vi "SDF Small Gasifier RT - Alarms.vi"() -> ()   [LabVIEW 2013]
uses:
  <vilib>/NI/Current Value Table/DataTypes/Boolean_Read.vi
  <vilib>/NI/Current Value Table/DataTypes/Double_Read.vi
  <vilib>/NI/Current Value Table/DataTypes/Boolean_Write.vi
  <vilib>/NI/Current Value Table/Type to Enum.vi
  <vilib>/NI/Current Value Table/DataTypes/Boolean_Type To Enum.vi
  <vilib>/NI/Current Value Table/DataTypes/Double_Type To Enum.vi
  <vilib>/NI/Current Value Table/FGVs/CVT Globals.vi
  <vilib>/NI/Current Value Table/FGVs/Tag Memory.vi
  <vilib>/NI/Current Value Table/Memory Block.vi
  <vilib>/NI/Current Value Table/DataTypes/Boolean_Memory Block.vi
  <vilib>/NI/Current Value Table/DataTypes/Double_Memory Block.vi
  <vilib>/NI/Current Value Table/Current Value Table.lvlib
panel:
  in  "Stop":bool
  out "Index":i32
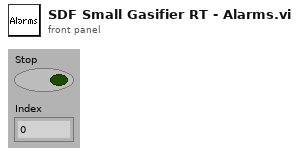
[diagram p1: front panel]
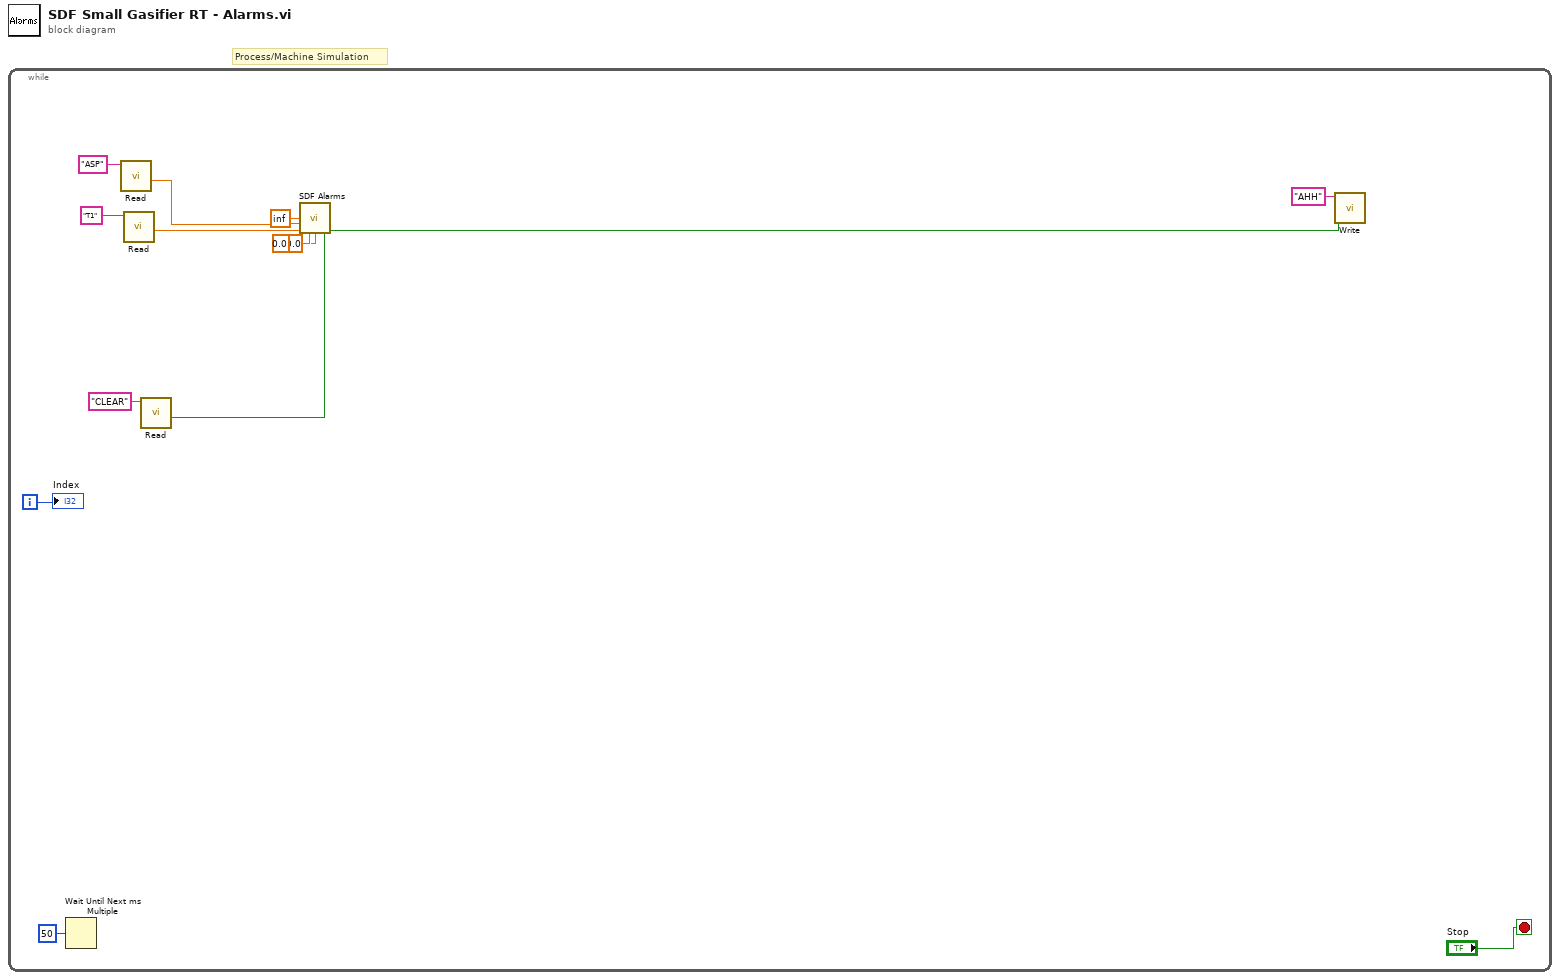
[diagram p0: block diagram]
diagram:
  # "Process/Machine Simulation"
  n1 = while {
    i -> [w13]
    stop <- "Stop" stop-if-true
    n2 = Wait Until Next ms Multiple(millisecond multiple=u32 50) -> ()  [unwired: 1 out]
    n3 = call-poly <vilib>:"Read.vi"("Tag Name"="ASP") -> ("Value"=w7:dbl)  [unwired: 9 in, 1 out]
    n4 = call-poly <vilib>:"Read.vi"("Tag Name"="T1") -> ("Value"=w6:dbl)  [unwired: 9 in, 1 out]
    n5 = call-poly <vilib>:"Read.vi"("Tag Name"="CLEAR") -> ("Value"=w5:bool)  [unwired: 9 in, 1 out]
    n6 = call "SDF Alarms.vi"("High High"=inf, "High"=w7, "LC-test"=w6, "LOW"=0.0, "LOW LOW"=0.0, "Reset"=w5) -> ("Warning"=w4:bool)  [unwired: 5 in, 4 out]
    n7 = call-poly <vilib>:"Write.vi"("Value"=w4, "Tag Name"="AHH") -> ()  [unwired: 9 in, 1 out]
    "Index" <- w13
  }
